vi "globalSetUp.vi"(8 "error in (no error)":errorcluster, 11 "testcase-CSMStatus in":refnum<class "testcase-CSMStatusStateRegisterUnregister.lvclass">) -> (0 "error out":errorcluster, 3 "testcase-CSMStatus out":refnum<class "testcase-CSMStatusStateRegisterUnregister.lvclass">)   [LabVIEW 2017, in "testcase-CSMStatusStateRegisterUnregister.lvclass"]
uses:
  testcase-CSMStatusStateRegisterUnregister.lvclass
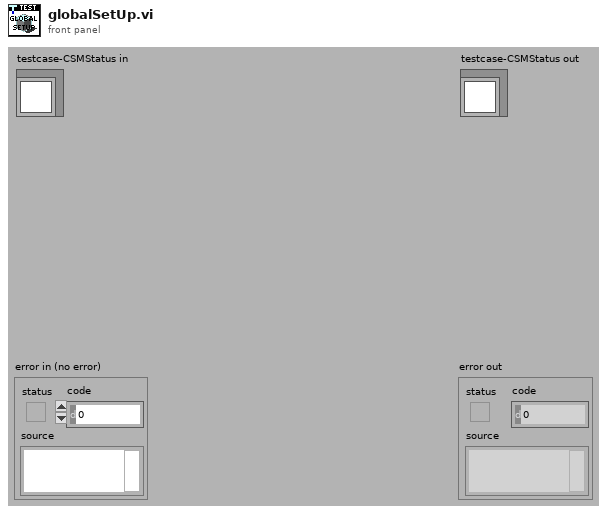
[diagram p1: front panel]
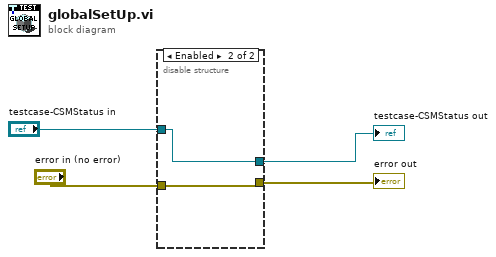
[diagram p0: block diagram]
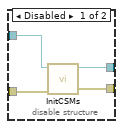
[diagram p2: hidden frame]
diagram:
  n1 = disable-structure shown="Enabled" {
    disable-tunnel: "error in (no error)" -> [w8 w9]
    disable-tunnel: [w7 w9] -> w3
    disable-tunnel: "testcase-CSMStatus in" -> [w6 w10]
    disable-tunnel: [w5 w10] -> w1
    frame Disabled {
      n2 = call "InitCSMs.vi"("error in"=w8, "testcase-CSMStatus in"=w6) -> ("error out"=w7:errorcluster, "testcase-CSMStatus out"=w5:refnum<class "testcase-CSMStatusStateRegisterUnregister.lvclass">)  [unwired: 8 in]
    }
    frame Enabled {
    }
  }
  "error out" <- w3
  "testcase-CSMStatus out" <- w1
